vi "Get Main Sequence Structure.vi"(8 "error in (no error)":errorcluster, 11 "Top Level Diagram":refnum<vi>) -> (0 "error out":errorcluster, 3 "Main.SeqStructure":refnum<vi>)   [LabVIEW 2015, in "Structures.lvclass"]
uses:
  Structures.lvclass
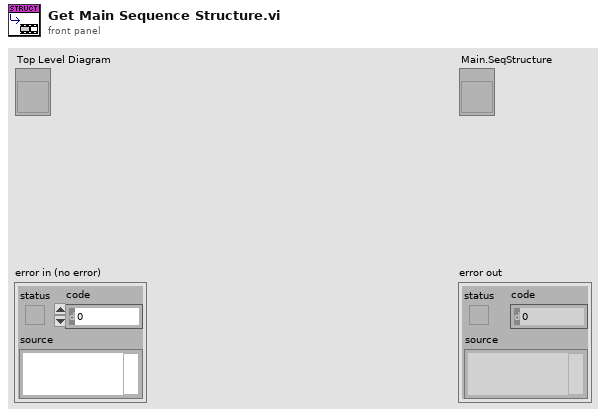
[diagram p1: front panel]
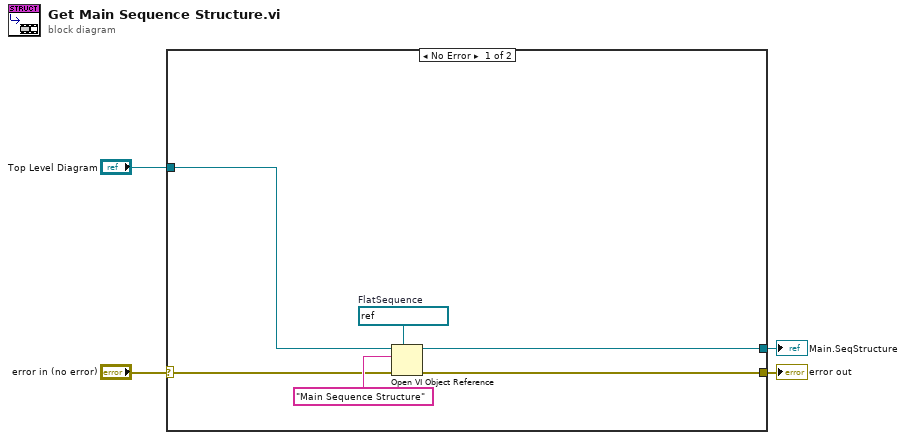
[diagram p0: block diagram]
diagram:
  n1 = case shown="No Error" "error in (no error)" {
    selector: "error in (no error)" -> [w7 w11]
    tunnel: [w6 w11] -> w3
    tunnel: "Top Level Diagram" -> [w8 _]
    tunnel: [w5 _] -> w1
    frame No Error {
      w9 = refnum<vi> refnum  # FlatSequence
      n2 = Open VI Object Reference(7:w9, 8:w7, 10:"Main Sequence Structure" ("name/order"), 11:w8) -> (0:w6:errorcluster, 3:w5:refnum<vi>)
    }
    frame Error {
    }
  }
  "error out" <- w3
  "Main.SeqStructure" <- w1
